vi "Reset.vi"(8 "error in (no error)":errorcluster, 11 "ATS9350 in":refnum<class "ATS9350.lvclass">) -> (0 "error out":errorcluster, 3 "ATS9350 out":refnum<class "ATS9350.lvclass">)   [LabVIEW 2015, in "ATS9350.lvclass"]
uses:
  ATS9350.lvclass
  ATS-VI/ATS_ctl/ATS_Async_Ctrl.ctl
  DAQ Class.lvclass
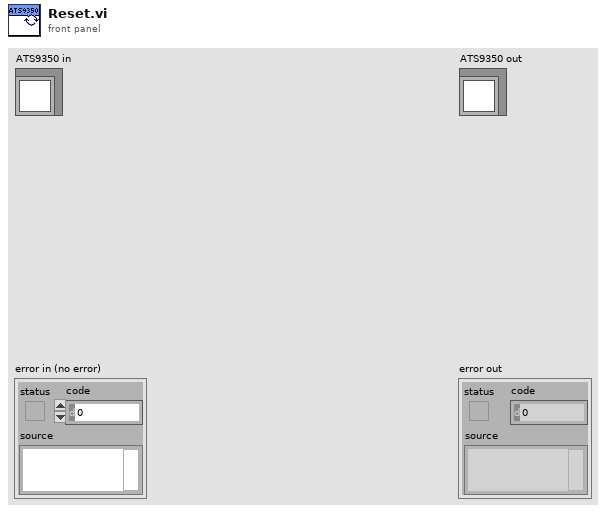
[diagram p1: front panel]
types:
  T1 = typedef "ATS_Async_Ctrl.ctl" = enum16{"SetupDMA", "StartCapture", "Get", "Get_Stream", "Abort", "Stop"}
  T2 = typedef "DAQ Class.lvclass/DAQ Parameters.ctl" = cluster{"Points Per A-Scan":u32, "A-Scans Per B-Scan":u32, "Number of B-Scans":u32, "B-Scans Per Transfer":u32, "Trigger Voltage":sgl, "Trigger Source":T3, "Trigger Slope":T4, "Channel":T5, "Clock":T6, "Bits per Sample":dbl, "Range":dbl, "Start Trim":u32, "Stop Trim":u32}
  T3 = typedef "DAQ Class.lvclass/Trigger Source.ctl" = enum16{"External", "Channel A", "Channel B"}
  T4 = typedef "DAQ Class.lvclass/Trigger Slope.ctl" = enum16{"Rising", "Falling"}
  T5 = typedef "OCT DAQ Channel Data Type.ctl" = enum16{"Channel 1", "Channel 2", "Channel 1 and 2"}
  T6 = typedef "DAQ Class.lvclass/Clock Control.ctl" = enum16{"Internal Clock", "External Clock"}
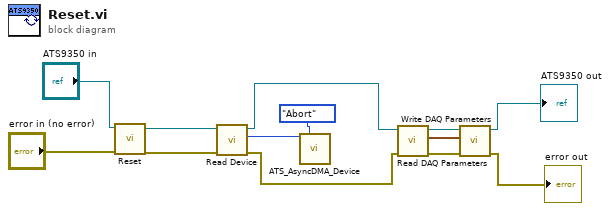
[diagram p0: block diagram]
diagram:
  n1 = call-parent "Reset.vi"("error in (no error)"="error in (no error)", "DAQ Class in"="ATS9350 in") -> ("error out"=w1:errorcluster, "DAQ Class out"=w2:refnum<class "ATS9350.lvclass">)  [unwired: 8 in]
  n2 = call-dynamic "Read Device.vi"("error in (no error)"=w1, "ATS9350 in"=w2) -> ("error out"=w8:errorcluster, "Device"=w10:i32, "ATS9350 out"=w9:refnum<class "ATS9350.lvclass">)  [unwired: 7 in]
  n3 = call "ATS_AsyncDMA_Device.vi"("DeviceIn"=w10, "ATS_Async_Ctrl"=ATS_Async_Ctrl."Abort") -> ()  [unwired: 9 in, 5 out]
  n4 = call-dynamic "Read DAQ Parameters.vi"("error in (no error)"=w8, "ATS9350 in"=w9) -> ("error out"=w5:errorcluster, "DAQ Parameters"=w6:T2, "ATS9350 out"=w7:refnum<class "ATS9350.lvclass">)  [unwired: 7 in]
  n5 = call-dynamic "Write DAQ Parameters.vi"("error in (no error)"=w5, "DAQ Parameters"=w6, "ATS9350 in"=w7) -> ("error out"=→"error out":errorcluster, "ATS9350 out"=→"ATS9350 out":refnum<class "ATS9350.lvclass">)  [unwired: 7 in]
